vi "反控参数变更.vi"(11 "设置参数":T1(ring)=enum."CODMn") -> ()   [LabVIEW 2016, in "斯坦道总磷总氮V2.lvlib"]
panel:
  in  "错误输入（无错误）":errorcluster
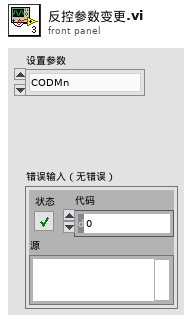
[diagram p1: front panel]
types:
  T1 = enum16{"", "CODMn", "PH", "氨氮", "总氮", "总磷", "CODCr", "电导率", "水温", "溶解氧", "浊度", "叶绿素", "藻密度", "ORP"}
  T2 = typedef "斯坦道总磷总氮V2.lvlib/量程设置.ctl" = enum32{"H", "L", "AUTO"}
  T3 = cluster{"水样测试量程模式":enum16{"H", "L", "AUTO"}, "空白核查量程模式":enum16{"H", "L", "AUTO"}, "跨度核查量程模式":enum16{"H", "L", "AUTO"}, "加标回收量程模式":enum16{"H", "L", "AUTO"}, "标样核查量程模式":enum16{"H", "L", "AUTO"}}
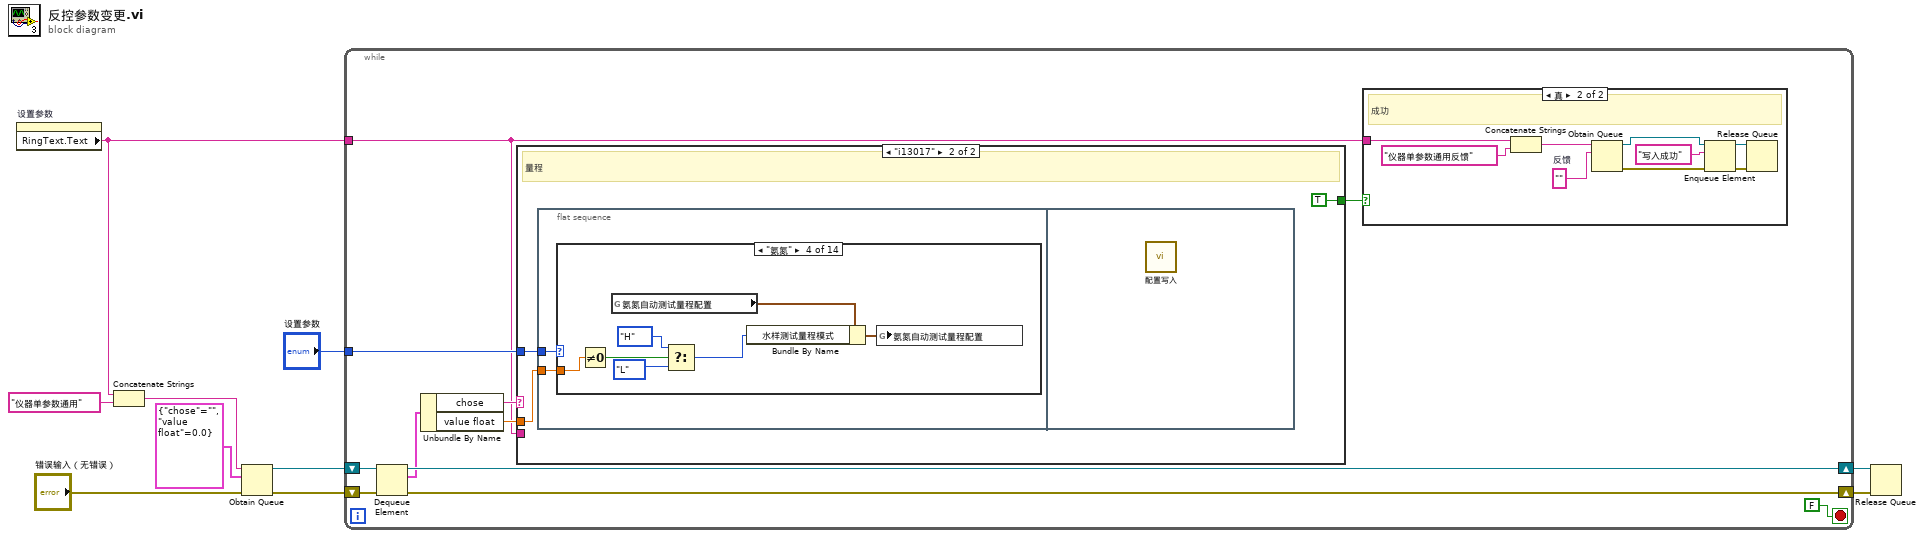
[diagram p0: block diagram]
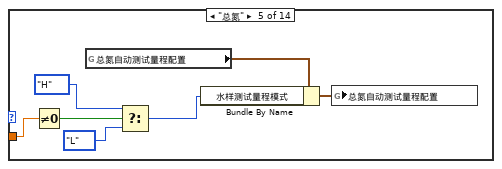
[diagram p7: hidden frame]
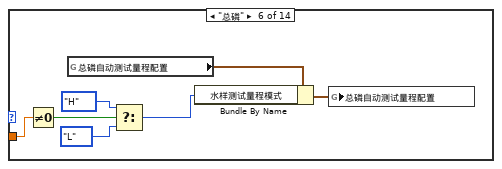
[diagram p8: hidden frame]
diagram:
  n1 = property on="设置参数" class="Enum (严格)"() -> ("RingText.Text"=w2:string)  [unwired: 2 in, 2 out]
  n2 = Concatenate Strings(w2, "仪器单参数通用" ("名称（未命名）")) -> (w7:string)
  n3 = Obtain Queue(name (unnamed)=w7, element data type=cluster{"chose":string, "value float":dbl} {"chose"="", "value float"=0.0}, error in (no error)="错误输入（无错误）") -> (queue out=w6:refnum<queue>, error out=w5:errorcluster)  [unwired: 2 in, 1 out]
  n4 = while {
    shift-right: [w19] -> w4
    shift-left: w6 -> [w21]
    shift-right: [w18] -> w3
    shift-left: w5 -> [w20]
    tunnel: w2 -> [w11]
    tunnel: "设置参数" -> [w12]
    stop <- FALSE stop-if-true
    n5 = Dequeue Element(queue=w21, error in (no error)=w20) -> (queue out=w19:refnum<queue>, element=w16:cluster{"chose":string, "value float":dbl}, error out=w18:errorcluster)  [unwired: 1 in, 1 out]
    n6 = Unbundle By Name(w16) -> ("chose"=w15:string, "value float"=w13:dbl)
    n7 = case shown="\"i13017\"" w15 {
      tunnel: w13 -> [_ w31]
      tunnel: [_ TRUE] -> w14
      tunnel: w12 -> [_ w32]
      tunnel: w11 -> [_ _]
      frame "假", Default {
      }
      frame "i13017" {
        # "量程"
        n8 = flat-sequence {
          tunnel: w32 -> [w35]
          tunnel: w31 -> [w34]
          frame #0 {
            n9 = case shown="\"氨氮\"" w35 {
              tunnel: w34 -> [_ _ _ w40 w47 w54 _ _ _ _ _ _ _ _]
              frame "", Default {
              }
              frame "CODMn" {
              }
              frame "PH" {
              }
              frame "氨氮" {
                n10 = Not Equal To 0?(x=w40) -> (x != 0?=w42:bool)
                n11 = global read "总磷总氮断电保存全局变量.vi" "氨氮自动测试量程配置"() -> (w38:T3)
                n12 = Select(t=量程设置."H" ("水样测试量程模式"), s=w42, f=量程设置."L" ("水样测试量程模式")) -> (s? t:f=w41:T2)
                n13 = Bundle By Name(cluster=w38, "水样测试量程模式"=w41) -> (w39:T3)
                n14 = global write "总磷总氮断电保存全局变量.vi" "氨氮自动测试量程配置"(w39) -> ()
              }
              frame "总氮" {
                n15 = Not Equal To 0?(x=w47) -> (x != 0?=w49:bool)
                n16 = global read "总磷总氮断电保存全局变量.vi" "总氮自动测试量程配置"() -> (w45:T3)
                n17 = Select(t=量程设置."H" ("水样测试量程模式"), s=w49, f=量程设置."L" ("水样测试量程模式")) -> (s? t:f=w48:T2)
                n18 = Bundle By Name(cluster=w45, "水样测试量程模式"=w48) -> (w46:T3)
                n19 = global write "总磷总氮断电保存全局变量.vi" "总氮自动测试量程配置"(w46) -> ()
              }
              frame "总磷" {
                n20 = Not Equal To 0?(x=w54) -> (x != 0?=w56:bool)
                n21 = global read "总磷总氮断电保存全局变量.vi" "总磷自动测试量程配置"() -> (w53:T3)
                n22 = Select(t=量程设置."H" ("水样测试量程模式"), s=w56, f=量程设置."L" ("水样测试量程模式")) -> (s? t:f=w55:T2)
                n23 = Bundle By Name(cluster=w53, "水样测试量程模式"=w55) -> (w52:T3)
                n24 = global write "总磷总氮断电保存全局变量.vi" "总磷自动测试量程配置"(w52) -> ()
              }
              frame "CODCr" {
              }
              frame "电导率" {
              }
              frame "水温" {
              }
              frame "溶解氧" {
              }
              frame "浊度" {
              }
              frame "叶绿素" {
              }
              frame "藻密度" {
              }
              frame "ORP" {
              }
            }
          }
          frame #1 {
            n25 = call "配置写入.vi"() -> ()  [unwired: 11 in, 1 out]
          }
        }
      }
    }
    n26 = case shown="真" w14 {
      tunnel: w11 -> [_ w29]
      frame False {
      }
      frame True {
        w24 = ""  # 反馈
        # "成功"
        n27 = Concatenate Strings(w29, "仪器单参数通用反馈" ("名称（未命名）")) -> (w23:string)
        n28 = Obtain Queue(name (unnamed)=w23, element data type=w24) -> (queue out=w25:refnum<queue>, error out=w26:errorcluster)  [unwired: 3 in, 1 out]
        n29 = Enqueue Element(queue=w25, element="写入成功" ("元素"), error in (no error)=w26) -> (queue out=w28:refnum<queue>, error out=w27:errorcluster)  [unwired: 1 in, 1 out]
        n30 = Release Queue(queue=w28, error in (no error)=w27) -> ()  [unwired: 1 in, 3 out]
      }
    }
  }
  n31 = Release Queue(queue=w4, error in (no error)=w3) -> ()  [unwired: 1 in, 3 out]
